vi "vision communication test vi.vi"() -> ()   [LabVIEW 2009]
panel:
  in  "y locations":i16[](array[numeric])
  in  "x locations":i16[](array[numeric])
  out "x out":i16[](array[numeric])
  out "y out":i16[](array[numeric])
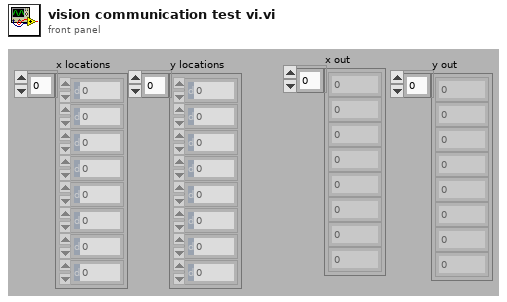
[diagram p1: front panel]
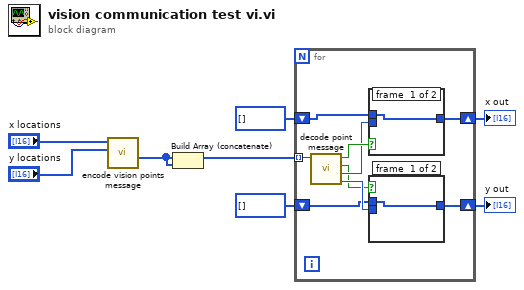
[diagram p0: block diagram]
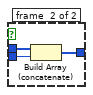
[diagram p2: hidden frame]
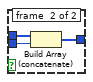
[diagram p3: hidden frame]
diagram:
  n1 = call "encode vision points message.vi"("y locations"="y locations", "x locations"="x locations") -> ("vision points message"=w2:u8[])  [unwired: 9 in]
  n2 = Build Array (concatenate)(w2, w2) -> (w1:u8[])
  n3 = for {
    tunnel: w1 -> [w17] mode=indexing
    shift-right: [w14] -> w5
    shift-left: i16[] [] -> [w13]
    shift-right: [w10] -> w6
    shift-left: i16[] [] -> [w9]
    n4 = call "decode point message.vi"("input stream"=w17) -> ("y value"=w12:i16, "x value"=w15:i16, "new y"=w11:bool, "new x"=w16:bool)  [unwired: 6 in, 1 out]
    n5 = case shown="True" w16 {
      tunnel: w15 -> [_ w25]
      tunnel: [w22 w24] -> w14
      tunnel: w13 -> [w22 w23]
      frame #0 {
      }
      frame #1 {
        n6 = Build Array (concatenate)(w23, w25) -> (w24:i16[])
      }
    }
    n7 = case shown="True" w11 {
      tunnel: w12 -> [_ w21]
      tunnel: [w18 w20] -> w10
      tunnel: w9 -> [w18 w19]
      frame #0 {
      }
      frame #1 {
        n8 = Build Array (concatenate)(w19, w21) -> (w20:i16[])
      }
    }
  }
  "y out" <- w6
  "x out" <- w5
